vi "Create General Tag.vi"(8 "error in (no error)":errorcluster, 11 "CVT Tags to Create":T1) -> (0 "error out":errorcluster, 3 "CVT Tags to Create":T1)   [LabVIEW 2016, in "CVT.lvlib"]
uses:
  CVT.lvlib
  <vilib>/NI/Current Value Table/Type Defs/File Format.ctl
  <vilib>/NI/Current Value Table/Type Defs/Single Tag.ctl
  <vilib>/NI/Current Value Table/Type Defs/Data Types.ctl
  <vilib>/NI/Current Value Table/Type Defs/Tag Grouping set.ctl
  <vilib>/NI/Current Value Table/Current Value Table.lvlib
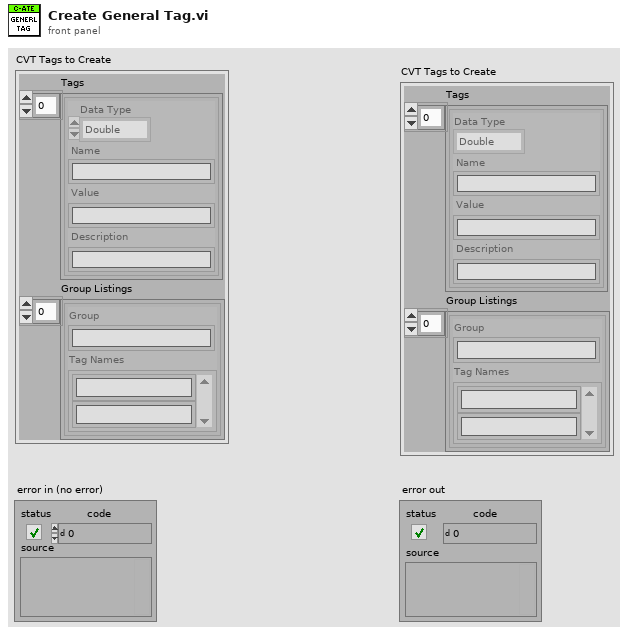
[diagram p1: front panel]
types:
  T1 = typedef "Current Value Table.lvlib/File Format.ctl" = cluster{"Tags":T2[], "Group Listings":T4[]}
  T2 = typedef "Current Value Table.lvlib/Single Tag.ctl" = cluster{"Data Type":T3, "Name":string, "Value":string, "Description":string}
  T3 = typedef "Current Value Table.lvlib/Data Types.ctl" = enum16{"Double", "Single", "I64", "I32", "I16", "I8", "U64", "U32", "U16", "U8", "String", "Boolean", "Array of U8", "Array of U16", "Array of U32", "Array of U64", "Array of I64", "Array of I32", "Array of I16", "Array of I8", "Array of Double", "Array of Single", "Array of Boolean", "Array of String"}
  T4 = typedef "Current Value Table.lvlib/Tag Grouping set.ctl" = cluster{"Group":string, "Tag Names":string[]}
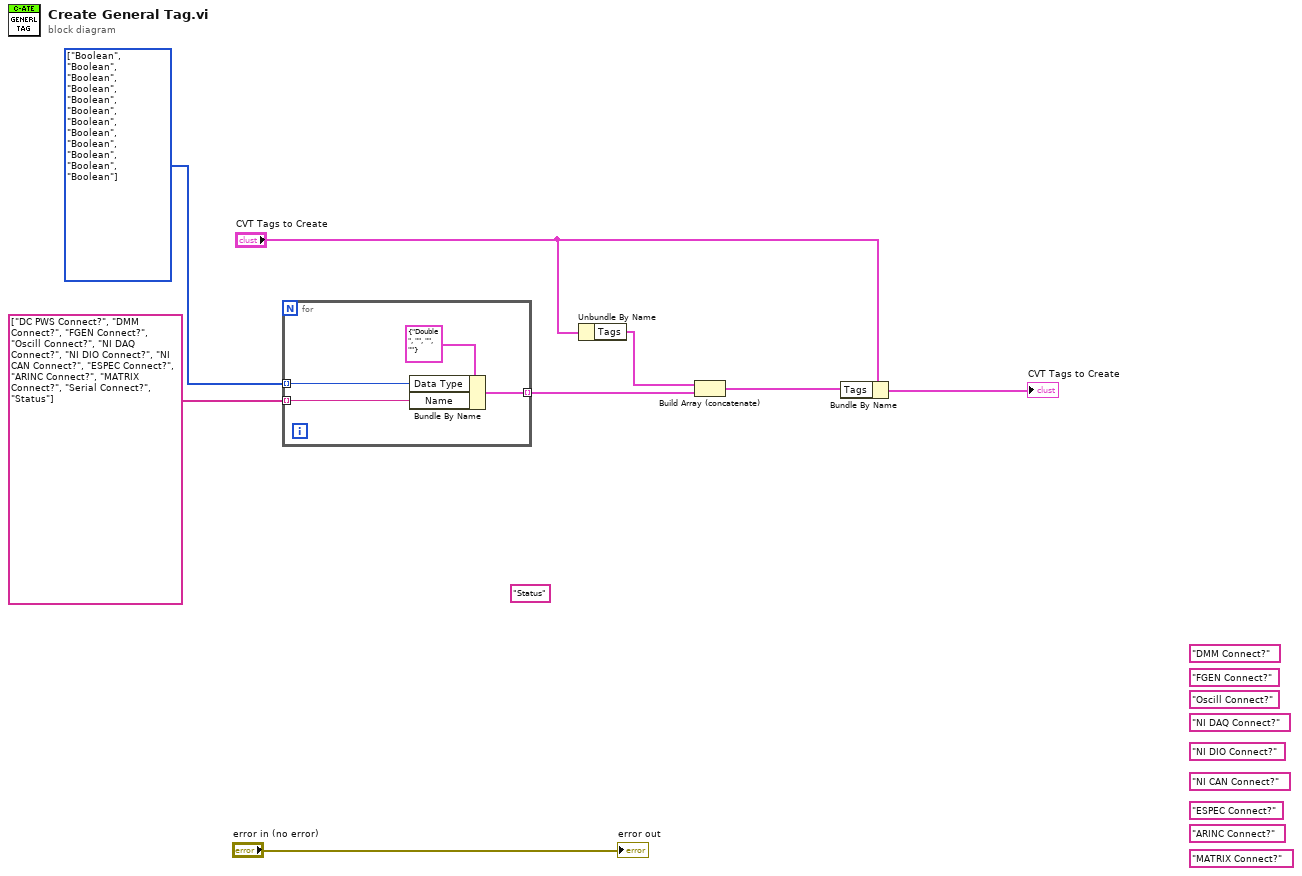
[diagram p0: block diagram]
diagram:
  w3 = T3[] [enum."Boolean", enum."Boolean", enum."Boolean", enum."Boolean", enum."Boolean", enum."Boolean", enum."Boolean", enum."Boolean", enum."Boolean", enum."Boolean", enum."Boolean", enum."Boolean"] items=["Double", "Single", "I64", "I32", "I16", "I8", "U64", "U32", "U16", "U8", "String", "Boolean", "Array of U8", "Array of U16", "Array of U32", "Array of U64", "Array of I64", "Array of I32", "Array of I16", "Array of I8", "Array of Double", "Array of Single", "Array of Boolean", "Array of String"] ("Array")
  (unwired) "Status"
  (unwired) "MATRIX Connect?" ("Tag Name")
  (unwired) "ARINC Connect?" ("Tag Name")
  (unwired) "ESPEC Connect?" ("Tag Name")
  (unwired) "NI CAN Connect?" ("Tag Name")
  (unwired) "NI DIO Connect?" ("Tag Name")
  (unwired) "NI DAQ Connect?" ("Tag Name")
  (unwired) "Oscill Connect?" ("Tag Name")
  (unwired) "FGEN Connect?" ("Tag Name")
  (unwired) "DMM Connect?" ("Tag Name")
  n1 = for {
    tunnel: string[] ["DC PWS Connect?", "DMM Connect?", "FGEN Connect?", "Oscill Connect?", "NI DAQ Connect?", "NI DIO Connect?", "NI CAN Connect?", "ESPEC Connect?", "ARINC Connect?", "MATRIX Connect?", "Serial Connect?", "Status"] -> [w12] mode=indexing
    tunnel: [w11] -> w6 mode=indexing
    tunnel: w3 -> [w9] mode=indexing
    n2 = Bundle By Name(cluster=T2 {"Data Type"=enum."Double", "Name"="", "Value"="", "Description"=""} ("Tag"), "Data Type"=w9, "Name"=w12) -> (w11:T2)
  }
  n3 = Unbundle By Name("CVT Tags to Create") -> ("Tags"=w4:T2[])
  n4 = Build Array (concatenate)(w4, w6) -> (w5:T2[])
  n5 = Bundle By Name(cluster="CVT Tags to Create", "Tags"=w5) -> (→"CVT Tags to Create":T1)
  "error out" <- "error in (no error)"
